vi "Query ProXR.vi"(8 "error in":errorcluster, 10 "Bytes to Read":u32, 11 "ProXR_IO in":refnum<class "ProXR.lvclass">) -> (0 "error out":errorcluster, 2 "Response":u8[](array[numeric]), 3 "ProXR_IO out":refnum<class "ProXR.lvclass">)   [LabVIEW 2019, in "ProXR.lvlib" / "ProXR.lvclass"]
uses:
  Library/ProXR.lvclass
  Library/ProXR.lvclass/ProXR.ctl
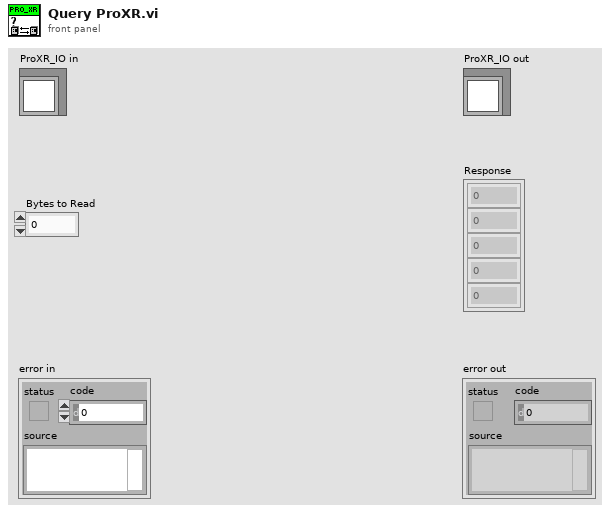
[diagram p1: front panel]
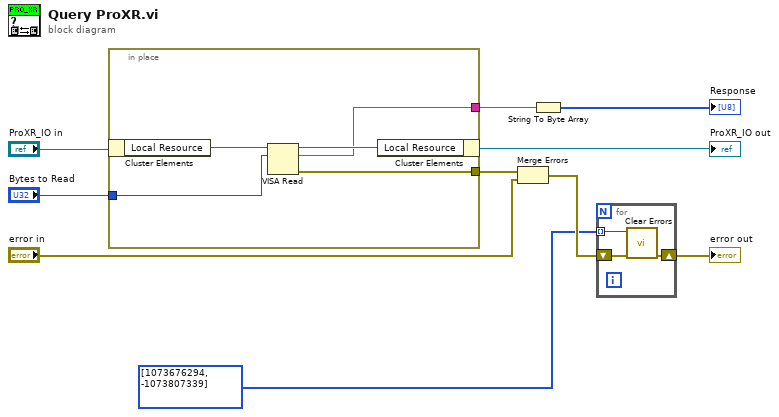
[diagram p0: block diagram]
diagram:
  n1 = in-place {
    in-place-border: [w14] -> w8
    in-place-border: [w13] -> w6
    in-place-border: "Bytes to Read" -> [w11]
    n2 = in-place-cluster #1("ProXR_IO in") -> ("Local Resource"=w12:refnum<visa-resource-name>)
    n3 = VISA Read(VISA resource name=w12, byte count=w11) -> (VISA resource name out=w15:refnum<visa-resource-name>, read buffer=w13:string, error out=w14:errorcluster)  [unwired: 1 in, 1 out]
    n4 = in-place-cluster #1("Local Resource"=w15) -> (→"ProXR_IO out":refnum<class "ProXR.lvclass">)
  }
  n5 = Merge Errors(w8, "error in") -> (w3:errorcluster)
  n6 = String To Byte Array(string=w6) -> (unsigned byte array=→"Response":u8[])
  n7 = for {
    shift-right: [w17] -> w2
    shift-left: w3 -> [w18]
    tunnel: i32[] [1073676294, -1073807339] -> [w16] mode=indexing
    n8 = call <vilib>:"Clear Errors.vi"("error in (no error)"=w18, "specific error code to clear (0: all)"=w16) -> ("error out"=w17:errorcluster)  [unwired: 4 in, 1 out]
  }
  "error out" <- w2
